vi "GET BLISS_Manage Persistent Data.vi"(7 "Action (Read)":T5=enum."Read Data", 8 "error in":errorcluster, 9 "Completed? (F)":bool, 11 "Data Parameters in":T1={"Server Index"=0, "username (e.g. name.i@pg.com)"="", "password"="", "Server Status List"=[], "search criteria"={"views"="", "reject codes"="", "sizes"="", "BLISS Image Types"=enum."Get Both PBQA And Reject Images", "Start Timestamp"=timestamp(0 s since 1904-01-01), "End Timesteamp"=timestamp(0 s since 1904-01-01), "# Images per folder"=1}, "PBQA File List"=[], "Reject File List"=[], "Save to Folder"=path "", "Server List"=[], "Start Time"=timestamp(0 s since 1904-01-01)} {"search criteria"."# Images per folder" min=1 max=10 step=1}) -> (0 "error out":errorcluster, 3 "Data Parameters Out":T1={"Server Index"=0, "username (e.g. name.i@pg.com)"="", "password"="", "Server Status List"=[], "search criteria"={"views"="", "reject codes"="", "sizes"="", "BLISS Image Types"=enum."Get Both PBQA And Reject Images", "Start Timestamp"=timestamp(0 s since 1904-01-01), "End Timesteamp"=timestamp(0 s since 1904-01-01), "# Images per folder"=1}, "PBQA File List"=[], "Reject File List"=[], "Save to Folder"=path "", "Server List"=[], "Start Time"=timestamp(0 s since 1904-01-01)} {"search criteria"."# Images per folder" min=1 max=10 step=1})   [LabVIEW 2018]
uses:
  Get BLISS_Global Variables.vi
  Get BLISS_Persistent Data Control.ctl
  Get BLISS_Index Control.ctl
  Get BLISS_Data Parameters.ctl
  Get BLISS_Server List 2.ctl
  Get BLISS_Search Criteria.ctl
  Get BLISS_Server Status List.ctl
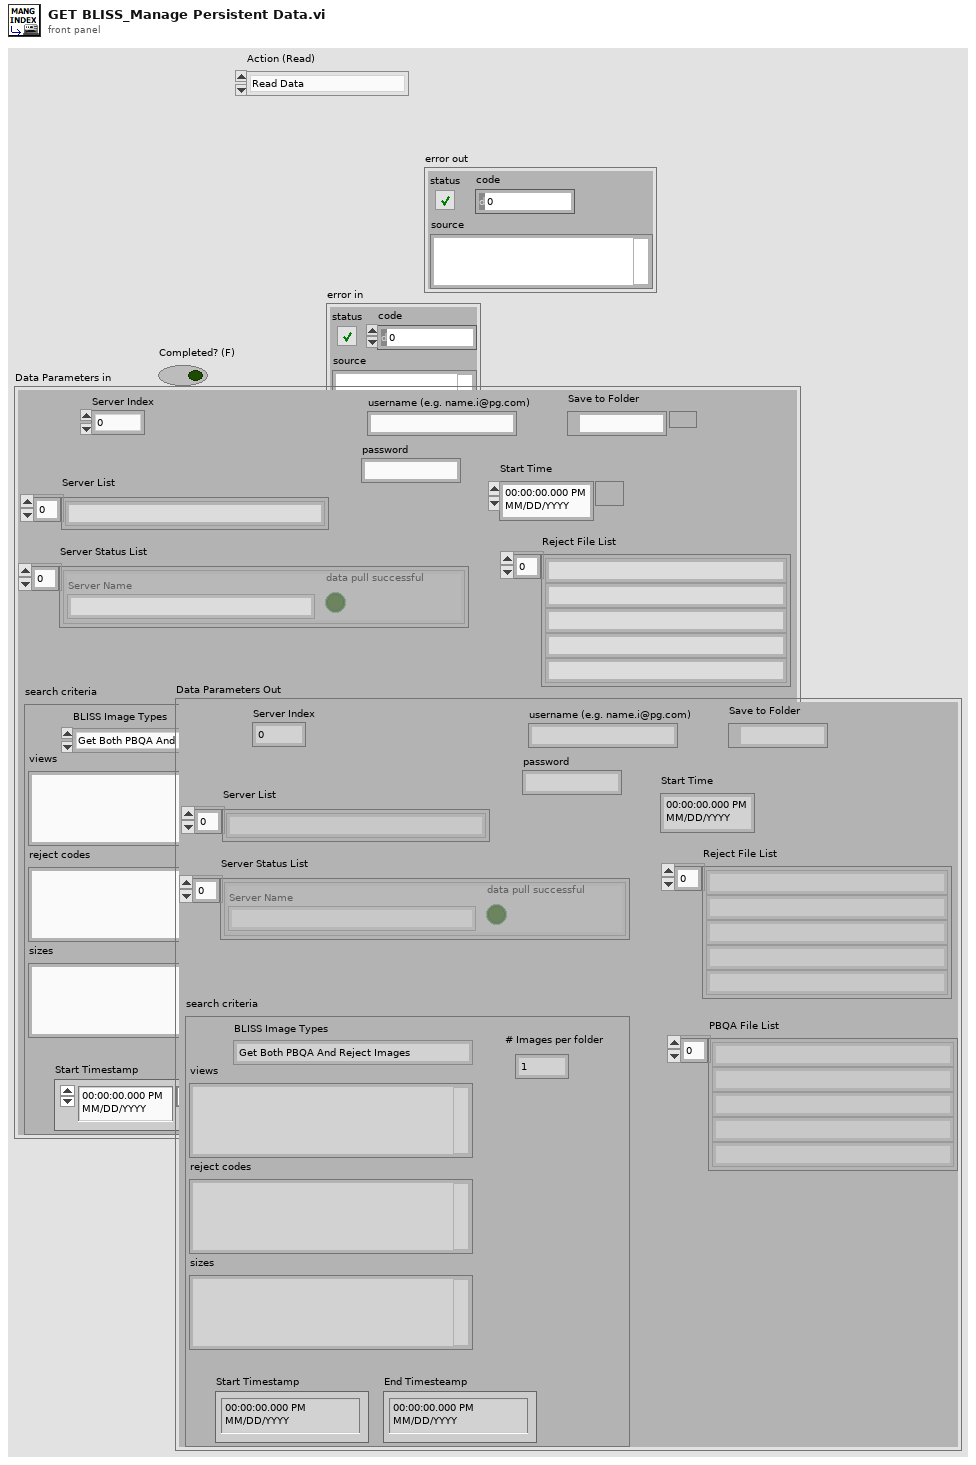
[diagram p1: front panel]
types:
  T1 = typedef "Get BLISS_Data Parameters.ctl" = cluster{"Server Index":i32, "username (e.g. name.i@pg.com)":string, "password":string, "Server Status List":T2, "search criteria":T4, "PBQA File List":string[], "Reject File List":string[], "Save to Folder":path, "Server List":string[], "Start Time":timestamp}
  T2 = typedef "Get BLISS_Server Status List.ctl" = T3[]
  T3 = typedef "Get BLISS_Server List 2.ctl" = cluster{"Server Name":string, "data pull successful":bool}
  T4 = typedef "Get BLISS_Search Criteria.ctl" = cluster{"views":string, "reject codes":string, "sizes":string, "BLISS Image Types":enum16{"Get Only Reject Images", "Get Only PBQA Images", "Get Both PBQA And Reject Images"}, "Start Timestamp":timestamp, "End Timesteamp":timestamp, "# Images per folder":i32}
  T5 = typedef "Get BLISS_Index Control.ctl" = enum16{"Save Data", "Read Data"}
  T6 = typedef "Get BLISS_Persistent Data Control.ctl" = cluster{"Server Index":i32, "Server List":cluster{"Server Name":string, "data pull successful":bool}[]}
  T7 = cluster{"Server Name":string, "data pull successful":bool}[]
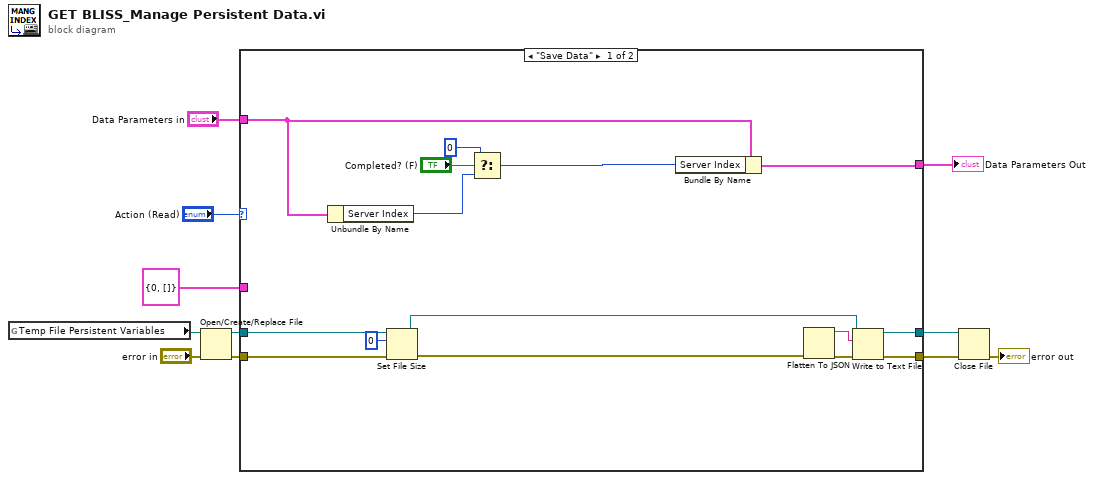
[diagram p0: block diagram]
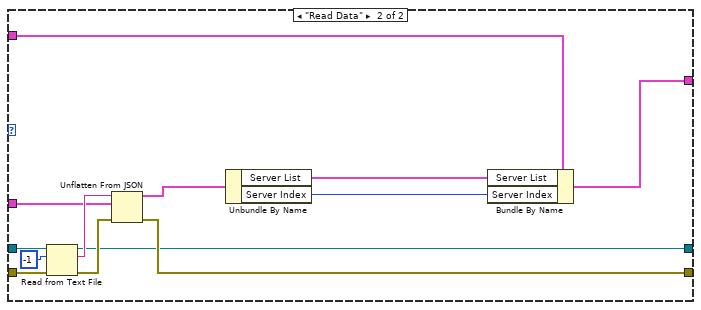
[diagram p2: hidden frame]
diagram:
  n1 = global read "Get BLISS_Global Variables.vi" "Temp File Persistent Variables"() -> (w7:path)
  n2 = Open/Create/Replace File(file path (use dialog)=w7, error in="error in") -> (refnum out=w8:refnum<file>, error out=w9:errorcluster)  [unwired: 4 in, 1 out]
  n3 = case shown="\"Save Data\"" "Action (Read)" {
    tunnel: [w18 w34] -> w11
    tunnel: [w19 w33] -> w10
    tunnel: w9 -> [w28 w40]
    tunnel: w8 -> [w26 w41]
    tunnel: "Data Parameters in" -> [w14 w32]
    tunnel: T6 {"Server Index"=0, "Server List"=[]} ("Persistent Data") -> [w22 w36]
    tunnel: [w12 w29] -> w1
    frame "Save Data" {
      n4 = Unbundle By Name(w14) -> ("Server Index"=w16:i32)
      n5 = Set File Size(4:w28, 6:i64 0 ("size (in bytes)"), 7:w26) -> (0:w24:errorcluster, 3:w25:refnum<file>)
      n6 = Select(t=0, s="Completed? (F)", f=w16) -> (s? t:f=w13:i32)
      n7 = Bundle By Name(cluster=w14, "Server Index"=w13) -> (w12:T1)
      n8 = Flatten To JSON(error in (no error)=w24) -> (anything=w21:cluster{}, JSON string=w20:string, 11:w23:errorcluster)  [unwired: 1 in]
      n9 = Write to Text File(file (use dialog)=w25, text=w20, error in=w23) -> (refnum out=w19:refnum<file>, error out=w18:errorcluster)  [unwired: 1 in, 1 out]
    }
    frame "Read Data" {
      n10 = Read from Text File(file (use dialog)=w41, count=-1, error in=w40) -> (refnum out=w33:refnum<file>, text=w37:string, error out=w38:errorcluster)  [unwired: 1 in, 1 out]
      n11 = Unflatten From JSON(JSON string=w37, type and defaults=w36, error in (no error)=w38) -> (value=w35:T6, error out=w34:errorcluster)  [unwired: 4 in]
      n12 = Unbundle By Name(w35) -> ("Server List"=w31:T7, "Server Index"=w30:i32)
      n13 = Bundle By Name(cluster=w32, "Server List"=w31, "Server Index"=w30) -> (w29:T1)
    }
  }
  "Data Parameters Out" <- w1
  n14 = Close File(refnum=w10, error in=w11) -> (error out=→"error out":errorcluster)  [unwired: 1 out]
